vi "_ADC_ Signal Downsample.vi"(6 "ADC Sampling Frequency Jitter":dbl, 7 "ADC Sampling Frequency":dbl, 9 "Input Wave":waveform(dbl)) -> (3 "Output Wave":waveform(dbl))   [LabVIEW 2014]
uses:
  <vilib>/measure/maresamp.llb/Resample Waveform (single shot).vi
  <vilib>/measure/NI_MAPro.lvlib
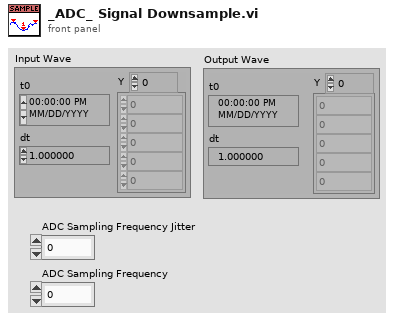
[diagram p1: front panel]
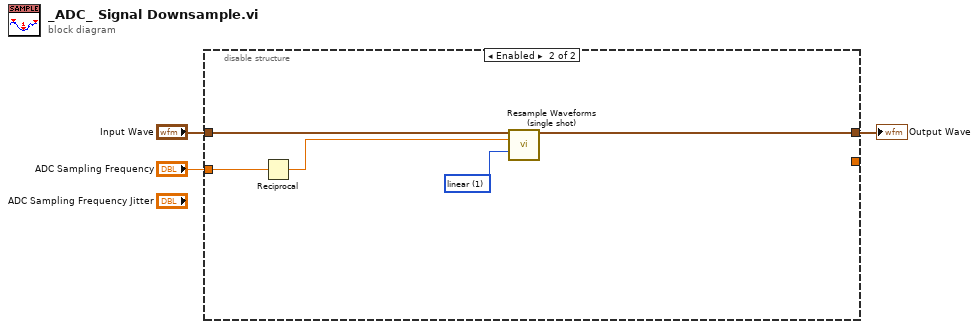
[diagram p0: block diagram]
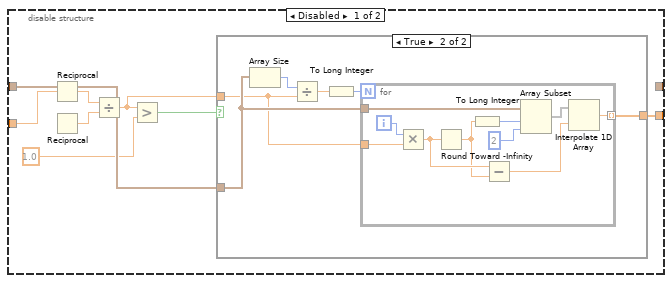
[diagram p2: hidden frame]
diagram:
  n1 = disable-structure shown="Enabled" {
    disable-tunnel: [w12 _] -> _
    disable-tunnel: "Input Wave" -> [w11 w34]
    disable-tunnel: "ADC Sampling Frequency" -> [w10 w33]
    disable-tunnel: [_ w31] -> w2
    frame Disabled {
      n2 = Reciprocal(x=w10) -> (1/x=w5:dbl)
      n3 = Reciprocal() -> (x=w9:dbl, 1/x=w4:dbl)
      n4 = Divide(x=w5, y=w4) -> (x/y=w8:dbl)
      n5 = Greater?(x=w8, y=1.0) -> (0:w6:bool)
      n6 = case shown="True" w6 {
        tunnel: [w13 w19] -> w12
        tunnel: w11 -> [w13 w18]
        tunnel: w8 -> [_ w17]
        frame False {
        }
        frame True {
          n7 = Array Size(array=w18) -> (size(s)=w14:i32)
          n8 = Divide(x=w14, y=w17) -> (x/y=w15:dbl)
          n9 = To Long Integer(number=w15) -> (32bit integer=w16:i32)
          n10 = for {
            N: w16 -> [_]
            tunnel: w18 -> [w27]
            tunnel: w17 -> [w28]
            tunnel: [w20] -> w19 mode=indexing
            i -> [w29]
            n11 = Multiply(x=w29, y=w28) -> (x*y=w23:dbl)
            n12 = Round Toward -Infinity(1:w23) -> (0:w22:dbl)
            n13 = To Long Integer(number=w22) -> (32bit integer=w26:i32)
            n14 = Subtract(x=w23, y=w22) -> (x-y=w21:dbl)
            n15 = Array Subset(array=w27, index=w26, length=2) -> (w24:void[])
            n16 = Interpolate 1D Array(1:w21, 2:w24) -> (0:w20:dbl)
          }
        }
      }
    }
    frame Enabled {
      w30 = u16 1 items=["coerce", "linear", "spline", "FIR filter"] ("interpolation mode")
      n17 = Reciprocal(x=w33) -> (1/x=w32:dbl)
      n18 = call-poly <vilib>:"Resample Waveforms (single shot).vi"("waveform in"=w34, "dt"=w32, "interpolation mode"=w30) -> ("resampled waveform out"=w31:waveform(dbl))  [unwired: 9 in, 3 out]
    }
  }
  "Output Wave" <- w2
